vi "ReverseDrive.vi"() -> ()   [LabVIEW 2013]
panel:
  in  "ReverseDrive?":bool
  out "Right":dbl
  out "Left":dbl
  in  "Right":dbl
  in  "Left":dbl
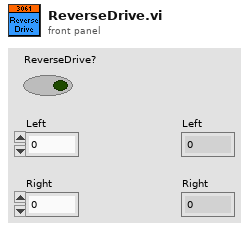
[diagram p1: front panel]
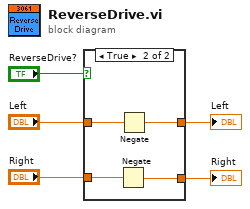
[diagram p0: block diagram]
diagram:
  n1 = case shown="True" "ReverseDrive?" {
    tunnel: [w7 w9] -> w3
    tunnel: "Left" -> [w7 w10]
    tunnel: [w6 w8] -> w1
    tunnel: "Right" -> [w6 w11]
    frame False {
    }
    frame True {
      n2 = Negate(x=w11) -> (-x=w8:dbl)
      n3 = Negate(x=w10) -> (-x=w9:dbl)
    }
  }
  "Left" <- w3
  "Right" <- w1
